vi "Test Get Parallel Tests Enabled.vi"(8 "error in (no error)":errorcluster, 11 "Configuration Manager Test in":refnum<class "Configuration Manager Test.lvclass">) -> (0 "error out":errorcluster, 3 "Configuration Manager Test out":refnum<class "Configuration Manager Test.lvclass">)   [LabVIEW 2020, in "Configuration Manager Test.lvclass"]
uses:
  Configuration Manager Test.lvclass
  Configuration Manager Test.lvclass/Configuration Manager Test.ctl
  source/User Interface/Configuration Manager/Configuration Manager.lvclass
  <vilib>/Astemes/LUnit/Test Case.lvclass
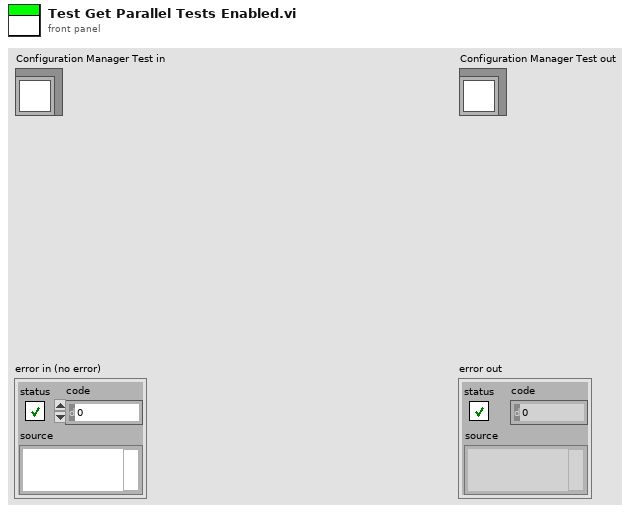
[diagram p1: front panel]
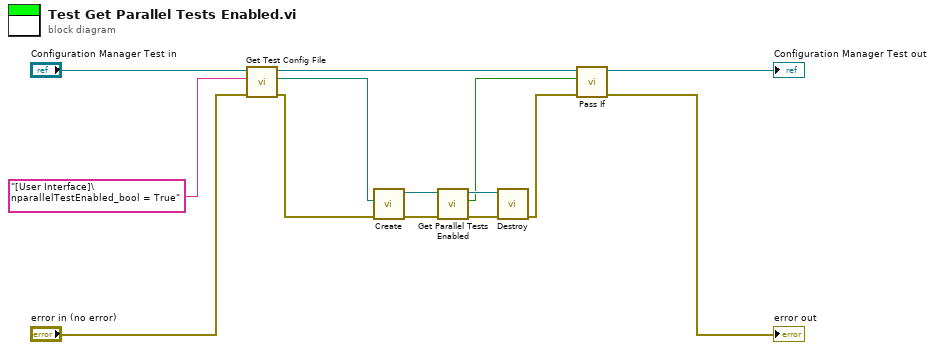
[diagram p0: block diagram]
diagram:
  n1 = call "Get Test Config File.vi"("error in (no error)"="error in (no error)", "File Content"="[User Interface]\nparallelTestEnabled_bool = True", "Configuration Manager Test in"="Configuration Manager Test in") -> ("error out"=w7:errorcluster, "File Path"=w1:path, "Configuration Manager Test out"=w4:refnum<class "Configuration Manager Test.lvclass">)  [unwired: 6 in]
  n2 = call "Create.vi"("error in (no error)"=w7, "configuration file path"=w1) -> ("error out"=w10:errorcluster, "Configuration Manager out"=w11:refnum<class "Configuration Manager.lvclass">)  [unwired: 8 in]
  n3 = call "Get Parallel Tests Enabled.vi"("error in (no error)"=w10, "Configuration Manager In"=w11) -> ("error out"=w8:errorcluster, "Parallel tetss enabled?"=w2:bool, "Configuration Manager Out"=w9:refnum<class "Configuration Manager.lvclass">)  [unwired: 7 in]
  n4 = call "Destroy.vi"("error in (no error)"=w8, "Configuration Manager In"=w9) -> ("error out"=w6:errorcluster)  [unwired: 9 in]
  n5 = call <vilib>:"Pass If.vi"("error in (no error)"=w6, "Pass?"=w2, "LUnit Test Case In"=w4) -> ("error out"=→"error out":errorcluster, "LUnit Test Case Out"=→"Configuration Manager Test out":refnum<class "Configuration Manager Test.lvclass">)  [unwired: 7 in]
